vi "DeleteRequestRow.vi"(8 "error in":errorcluster, 10 "RequestID":u32) -> (0 "error out":errorcluster)   [LabVIEW 2015]
uses:
  TypeDef/RequestsTableDbTableName.ctl
  <vilib>/addons/database/Connection.llb/DB Tools Open Connec (Path).vi
  <vilib>/addons/database/NI_Database_API.lvlib
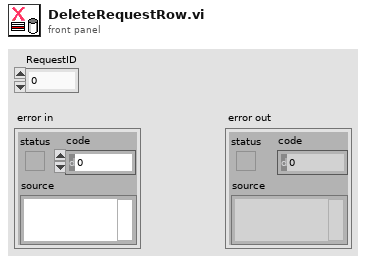
[diagram p1: front panel]
types:
  T1 = typedef "RequestsTableDbTableName.ctl" = string
  T2 = typedef "NI_Database_API.lvlib/Conn ObjectReference.ctl" = refnum<k1>
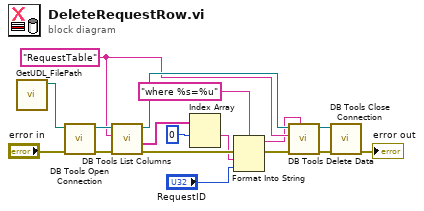
[diagram p0: block diagram]
diagram:
  w7 = T1 "RequestTable" ("table")
  n1 = call "GetUDL_FilePath.vi"() -> ("UDL file path"=w17:path)  [unwired: 11 in]
  n2 = call-poly <vilib>:"DB Tools Open Connection.vi"("error in (no error)"="error in", "connection information"=w17) -> ("error out"=w14:errorcluster, "connection reference"=w10:T2)  [unwired: 6 in]
  n3 = call <vilib>:"DB Tools List Columns.vi"("error in (no error)"=w14, "table"=w7, "connection reference"=w10) -> ("error out"=w11:errorcluster, "columns"=w8:string[], "connection reference out"=w9:T2)  [unwired: 1 in, 1 out]
  n4 = Index Array(array=w8, index #1=0 ("index")) -> (element #1=w5:string)  [unwired: 1 in, 1 out]
  n5 = Format Into String(format string="where %s=%u", error in=w11, w5, "RequestID") -> (resulting string=w1:string, error out=w2:errorcluster)  [unwired: 1 in]
  n6 = call <vilib>:"DB Tools Delete Data.vi"("condition"=w1, "error in (no error)"=w2, "table"=w7, "connection reference"=w9) -> ("error out"=w13:errorcluster, "connection reference out"=w12:T2)  [unwired: 6 in]
  n7 = call <vilib>:"DB Tools Close Connection.vi"("error in (no error)"=w13, "connection reference"=w12) -> ("error out"=→"error out":errorcluster)  [unwired: 5 in]
